vi "TrasportParameterInit.vi"(8 "error in (no error)":errorcluster, 11 "Position":T1[](array[typedef])) -> (0 "Error Out":errorcluster)   [LabVIEW 2016, in "SeqProcessor.lvlib"]
uses:
  SeqProcessor.lvlib
  Parameter/controls/Position.ctl
  Parameter/Parameter.lvlib
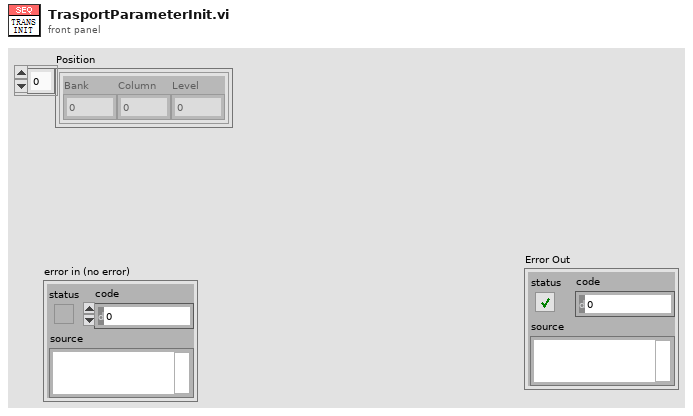
[diagram p1: front panel]
types:
  T1 = typedef "Parameter.lvlib/Position.ctl" = cluster{"Bank":u8, "Column":u8, "Level":u8}
  T2 = typedef "Parameter.lvlib/StockerInfo.ctl" = cluster{"Bank":u8, "Level":u8, "Column":u8, "RotateHPPosition":dbl, "RotateOPPosition":dbl, "LiftUpperLimit":dbl, "LiftLowerLimit":dbl, "ForkOPPositon1":dbl, "ForkOPPosition2":dbl, "TravelLimit":T3, "LiftLimit":T3, "RotateLimit":T3, "ForkLimit":T3}
  T3 = typedef "Parameter.lvlib/LimitPosition.ctl" = cluster{"HPES":dbl, "OPES":dbl}
  T4 = typedef "Parameter.lvlib/CasstteCoordinate.ctl" = cluster{"Travel":dbl, "Lift":dbl, "Upper":dbl, "Lower":dbl}
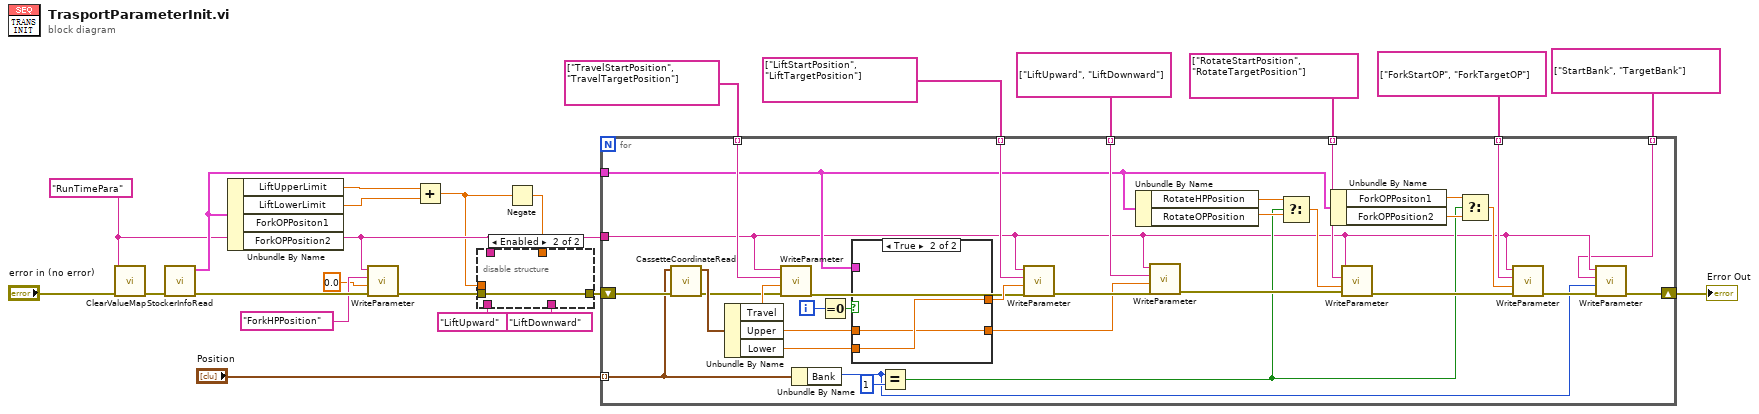
[diagram p0: block diagram]
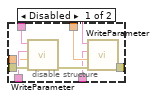
[diagram p2: hidden frame]
diagram:
  w10 = "RunTimePara" ("MapName")
  n1 = call "ClearValueMap.vi"("error in (no error)"="error in (no error)", "MapName"=w10) -> ("error out"=w19:errorcluster)  [unwired: 8 in, 1 out]
  n2 = call "StockerInfoRead.vi"("error in (no error)"=w19) -> ("Error Out"=w18:errorcluster, "StockerInfo"=w17:T2)  [unwired: 8 in, 1 out]
  n3 = Unbundle By Name(w17) -> ("LiftUpperLimit"=w15:dbl, "LiftLowerLimit"=w14:dbl)  [unwired: 2 out]
  n4 = call "WriteParameter.vi"("error in (no error)"=w18, "Value"=0.0, "Parameter"="ForkHPPosition", "MapName"=w10) -> ("Error Out"=w2:errorcluster)  [unwired: 6 in, 1 out]
  n5 = Add(x=w15, y=w14) -> (x+y=w9:dbl)
  n6 = Negate(x=w9) -> (-x=w8:dbl)
  n7 = disable-structure shown="Enabled" {
    disable-tunnel: [w31 w32] -> w13
    disable-tunnel: w2 -> [w30 w32]
    disable-tunnel: "LiftUpward" ("Parameter") -> [w28 _]
    disable-tunnel: w10 -> [w27 _]
    disable-tunnel: w9 -> [w26 _]
    disable-tunnel: w8 -> [w25 _]
    disable-tunnel: "LiftDownward" ("Parameter") -> [w24 _]
    frame Disabled {
      n8 = call "WriteParameter.vi"("error in (no error)"=w30, "Value"=w26, "Parameter"=w28, "MapName"=w27) -> ("Error Out"=w29:errorcluster)  [unwired: 6 in, 1 out]
      n9 = call "WriteParameter.vi"("error in (no error)"=w29, "Value"=w25, "Parameter"=w24, "MapName"=w27) -> ("Error Out"=w31:errorcluster)  [unwired: 6 in, 1 out]
    }
    frame Enabled {
    }
  }
  n10 = for {
    tunnel: w10 -> [w35]
    shift-right: [w36] -> w6
    shift-left: w13 -> [w60]
    tunnel: string[] ["TravelStartPosition", "TravelTargetPosition"] -> [w58] mode=indexing
    tunnel: string[] ["LiftStartPosition", "LiftTargetPosition"] -> [w53] mode=indexing
    tunnel: string[] ["RotateStartPosition", "RotateTargetPosition"] -> [w52] mode=indexing
    tunnel: "Position" -> [w51] mode=indexing
    tunnel: w17 -> [w42]
    tunnel: string[] ["LiftUpward", "LiftDownward"] -> [w46] mode=indexing
    tunnel: string[] ["ForkStartOP", "ForkTargetOP"] -> [w43] mode=indexing
    tunnel: string[] ["StartBank", "TargetBank"] -> [w34] mode=indexing
    i -> [w56]
    n11 = call "CassetteCoordinateRead.vi"("error in (no error)"=w60, "Position"=w51) -> ("error out"=w59:errorcluster, "Coordinate"=w66:T4)  [unwired: 8 in]
    n12 = Unbundle By Name(w66) -> ("Travel"=w65:dbl, "Upper"=w55:dbl, "Lower"=w49:dbl)
    n13 = call "WriteParameter.vi"("error in (no error)"=w59, "Value"=w65, "Parameter"=w58, "MapName"=w35) -> ("Error Out"=w50:errorcluster)  [unwired: 6 in, 1 out]
    n14 = Unbundle By Name(w51) -> ("Bank"=w33:u8)
    n15 = Equal To 0?(x=w56) -> (x = 0?=w57:bool)
    n16 = case shown="True" w57 {
      tunnel: w55 -> [w68 w69]
      tunnel: w42 -> [_ _]
      tunnel: [w68 w70] -> w54
      tunnel: w49 -> [w67 w70]
      tunnel: [w67 w69] -> w45
      frame False {
      }
      frame True {
      }
    }
    n17 = Equal?(x=w33, y=u8 1) -> (x = y?=w38:bool)
    n18 = call "WriteParameter.vi"("error in (no error)"=w50, "Value"=w54, "Parameter"=w53, "MapName"=w35) -> ("Error Out"=w48:errorcluster)  [unwired: 6 in, 1 out]
    n19 = Unbundle By Name(w42) -> ("RotateHPPosition"=w64:dbl, "RotateOPPosition"=w63:dbl)
    n20 = call "WriteParameter.vi"("error in (no error)"=w48, "Value"=w45, "Parameter"=w46, "MapName"=w35) -> ("Error Out"=w47:errorcluster)  [unwired: 6 in, 1 out]
    n21 = Select(t=w64, s=w38, f=w63) -> (s? t:f=w62:dbl)
    n22 = Unbundle By Name(w42) -> ("ForkOPPositon1"=w40:dbl, "ForkOPPosition2"=w41:dbl)
    n23 = call "WriteParameter.vi"("error in (no error)"=w47, "Value"=w62, "Parameter"=w52, "MapName"=w35) -> ("Error Out"=w44:errorcluster)  [unwired: 6 in, 1 out]
    n24 = Select(t=w40, s=w38, f=w41) -> (s? t:f=w39:dbl)
    n25 = call "WriteParameter.vi"("error in (no error)"=w44, "Value"=w39, "Parameter"=w43, "MapName"=w35) -> ("Error Out"=w37:errorcluster)  [unwired: 6 in, 1 out]
    n26 = call "WriteParameter.vi"("error in (no error)"=w37, "Value"=w33, "Parameter"=w34, "MapName"=w35) -> ("Error Out"=w36:errorcluster)  [unwired: 6 in, 1 out]
  }
  "Error Out" <- w6
